vi "make scan analysis files.vi"(8 "error in (no error)":errorcluster, 9 "<scan number>":i32, 10 "<Scans Path>":path, 11 "<ScanInfo FIle path>":path) -> (0 "error out":errorcluster)   [LabVIEW 2018]
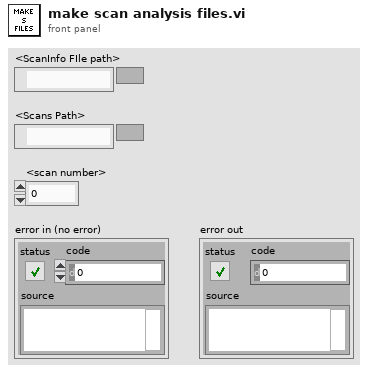
[diagram p1: front panel]
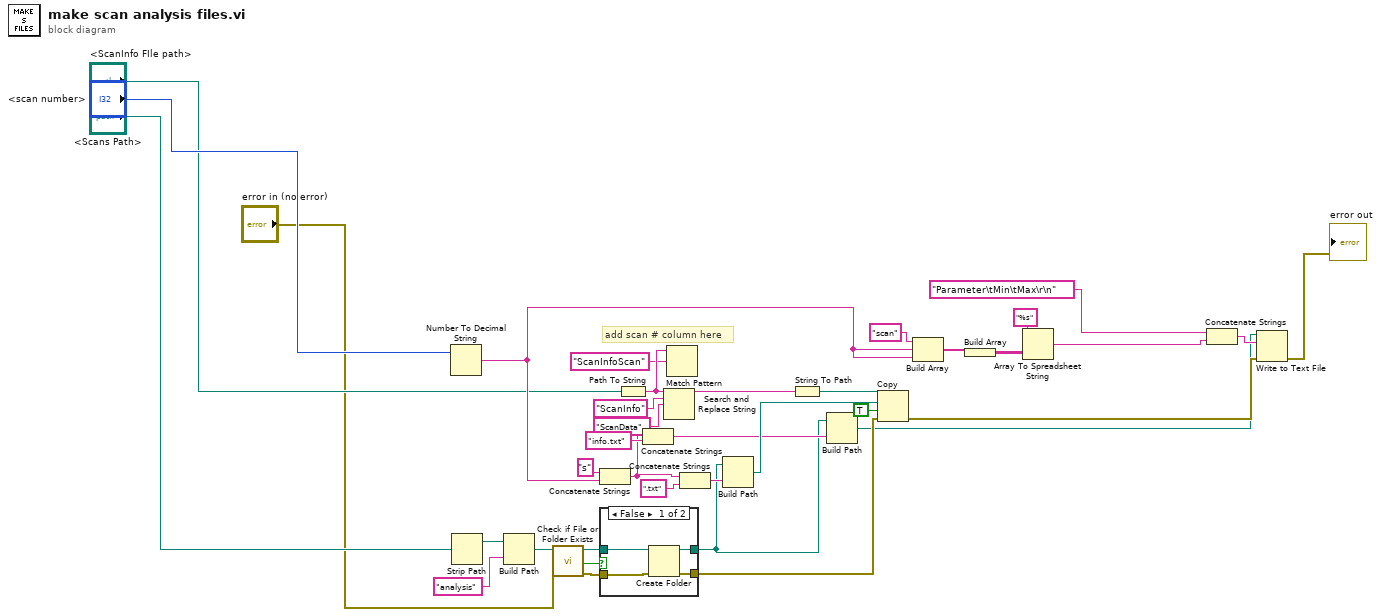
[diagram p0: block diagram]
diagram:
  # "add scan # column here"
  n1 = Number To Decimal String(number="<scan number>") -> (decimal integer string=w36:string)  [unwired: 1 in]
  n2 = Strip Path(path="<Scans Path>") -> (stripped path=w24:path)  [unwired: 1 out]
  n3 = Build Path(base path=w24, name or relative path="analysis") -> (appended path=w14:path)
  n4 = call <vilib>:"Check if File or Folder Exists.vi"("error in (no error)"="error in (no error)", "path"=w14) -> ("error out"=w30:errorcluster, "file or folder exists?"=w13:bool, "dup path"=w12:path)  [unwired: 7 in]
  n5 = Concatenate Strings("s" ("string"), w36) -> (w1:string)
  n6 = case shown="False" w13 {
    tunnel: w12 -> [w41 w43]
    tunnel: [w40 w43] -> w2
    tunnel: w30 -> [w39 w42]
    tunnel: [w38 w42] -> w31
    frame False {
      n7 = Create Folder(path (use dialog)=w41, error in=w39) -> (created path=w40:path, error out=w38:errorcluster)  [unwired: 1 in, 1 out]
    }
    frame True {
    }
  }
  n8 = Path To String(path="<ScanInfo FIle path>") -> (string=w18:string)
  n9 = Concatenate Strings(w1, "info.txt" ("string")) -> (w3:string)
  n10 = Search and Replace String(input string=w18, search string="ScanInfo" ("replace string (\"\")"), replace string="ScanData" ("search string")) -> (result string=w20:string)  [unwired: 5 in, 3 out]
  n11 = Match Pattern(string=w18, regular expression="ScanInfoScan" ("replace string (\"\")")) -> ()  [unwired: 1 in, 4 out]
  n12 = Concatenate Strings(w1, ".txt" ("string")) -> (w16:string)
  n13 = Build Path(base path=w2, name or relative path=w16) -> (appended path=w15:path)
  n14 = String To Path(string=w20) -> (path=w19:path)
  n15 = Build Path(base path=w2, name or relative path=w3) -> (appended path=w5:path)
  n16 = Copy(8:w31, 9:TRUE ("overwrite (F)"), 10:w15, 11:w19) -> (0:w32:errorcluster)  [unwired: 1 in, 2 out]
  n17 = Build Array("scan" ("name or relative path"), w36, w36) -> (w10:string[])
  n18 = Build Array(w10) -> (w9:string[][])
  n19 = Array To Spreadsheet String(array=w9, 3:"%s" ("format string")) -> (spreadsheet string=w6:string)  [unwired: 1 in]
  n20 = Concatenate Strings("Parameter\tMin\tMax\r\n" ("name or relative path"), w6) -> (w28:string)
  n21 = Write to Text File(file (use dialog)=w5, text=w28, error in=w32) -> (error out=→"error out":errorcluster)  [unwired: 1 in, 2 out]
